vi "DAC Run.vi"(8 "error in":errorcluster, 11 "DAC HeatFlow AOV in":refnum<class "DAC HeatFlow AOV.lvclass">) -> (0 "error out":errorcluster, 3 "DAC HeatFlow AOV out":refnum<class "DAC HeatFlow AOV.lvclass">)   [LabVIEW 2019, in "DAC.lvlib" / "DAC HeatFlow AOV.lvclass"]
uses:
  DAC HeatFlow AOV.lvclass
  C:/Users/krio/Documents/LV_Projects/test-stand/App/DAC/DAC.lvclass
  DAC.lvclass/DAC.ctl
  DAC HeatFlow AOV.lvclass/DAC HeatFlow AOV.ctl
  <vilib>/DAQmx/read.llb/DAQmx Read (Analog Wfm 1Chan NSamp).vi
  <vilib>/Analysis/baseanly.llb/Mean (DBL).vi
  <vilib>/DAQmx/miscellaneous.llb/DAQmx Fill In Error Info.vi
  DAC.lvclass
  <vilib>/Analysis/NI_AALBase.lvlib
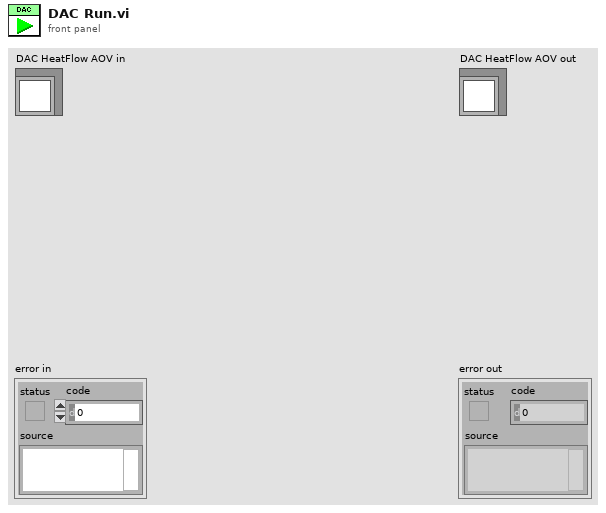
[diagram p1: front panel]
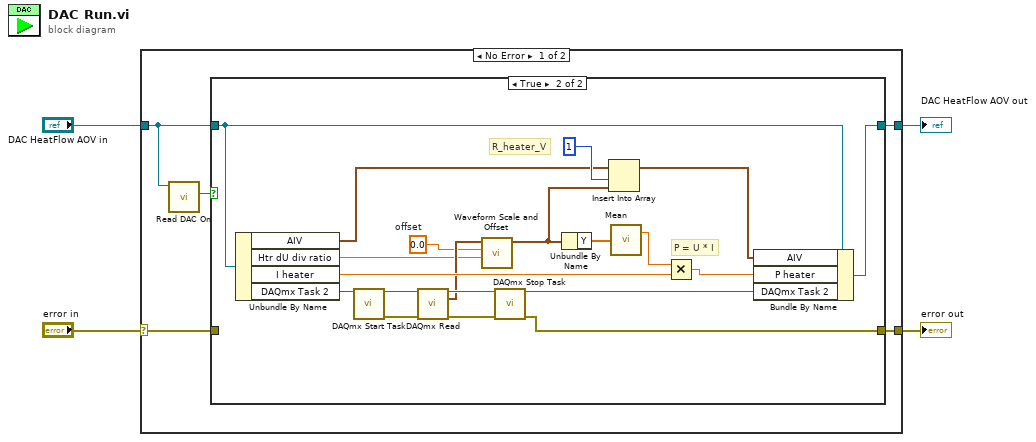
[diagram p0: block diagram]
diagram:
  n1 = case shown="No Error" "error in" {
    selector: "error in" -> [w7 w33]
    tunnel: [w6 w33] -> w2
    tunnel: [w8 w32] -> w1
    tunnel: "DAC HeatFlow AOV in" -> [w5 w32]
    frame No Error {
      n2 = call "Read DAC On.vi"("DAC in"=w5) -> ("DAC On"=w9:bool)  [unwired: 8 in, 2 out]
      n3 = case shown="True" w9 {
        tunnel: w5 -> [w11 w24]
        tunnel: [w11 w26] -> w8
        tunnel: w7 -> [w10 _]
        tunnel: [w10 w19] -> w6
        frame False {
        }
        frame True {
          w14 = 0.0  # offset
          # "P = U * I"
          # "R_heater_V"
          n4 = Unbundle By Name(w24) -> ("AIV"=w17:waveform(dbl)[], "Htr dU div ratio"=w15:dbl, "I heater"=w18:dbl, "DAQmx Task 2"=w31:refnum<k21>)
          n5 = call <vilib>:"DAQmx Start Task.vi"("task/channels in"=w31) -> ("task out"=w30:refnum<k21>, "error out"=w28:errorcluster)  [unwired: 13 in]
          n6 = call-poly <vilib>:"DAQmx Read.vi"("task/channels in"=w30, "error in"=w28) -> ("task out"=w29:refnum<k21>, "data"=w16:waveform(dbl), "error out"=w27:errorcluster)  [unwired: 11 in]
          n7 = call <vilib>:"Waveform Scale and Offset.vi"("scale"=w15, "offset"=w14, "waveform in"=w16) -> ("waveform out"=w12:waveform(dbl))  [unwired: 7 in, 1 out]
          n8 = call <vilib>:"DAQmx Stop Task.vi"("task/channels in"=w29, "error in"=w27) -> ("task out"=w25:refnum<k21>, "error out"=w19:errorcluster)  [unwired: 12 in]
          n9 = Unbundle By Name(w12) -> ("Y"=w22:dbl[])
          n10 = Insert Into Array "Insert Into Array"(array=w17, index=1, new element=w12) -> (w20:waveform(dbl)[])
          n11 = call-poly <vilib>:"Mean.vi"("X"=w22) -> ("mean"=w13:dbl)  [unwired: 1 out]
          n12 = Multiply(x=w13, y=w18) -> (x*y=w21:dbl)
          n13 = Bundle By Name(cluster=w24, "AIV"=w20, "P heater"=w21, "DAQmx Task 2"=w25) -> (w26:refnum<class "DAC HeatFlow AOV.lvclass">)
        }
      }
    }
    frame Error {
    }
  }
  "error out" <- w2
  "DAC HeatFlow AOV out" <- w1
